vi "Calibrator Panel.vi"(8 "error in (no error)":errorcluster, 11 "Varian Magnet.lvclass In":refnum<class "Varian Magnet.lvclass">) -> (0 "error out":errorcluster, 3 "Varian Magnet.lvclass Out":refnum<class "Varian Magnet.lvclass">)   [LabVIEW 2009, in "Varian Magnet.lvclass"]
doc: "This is a low level control panel for the Varian magnet. It allows for reading and setting of the control voltage and displays the raw hall voltage. It also contains functions for calibrating various features of the magnet program."
uses:
  Varian Magnet.lvclass
  <vilib>/gmath/interp.llb/in_piecewise interp poly control.ctl
  Varian Magnet.lvclass/Varian Magnet.ctl
  <vilib>/Utility/file.llb/Write To Spreadsheet File (DBL).vi
  Varian/Varian.lvlib
  Fluke Multimeter/Fluke Multimeter.lvclass
  <vilib>/gmath/NI_Gmath.lvlib
panel:
  out "extrapolated":T1 {"x locations" format="%.4g"; "coefficients" format="%.4g"}
  in  "Write Current Calibration\nto Long-Term Calibration":bool
  in  "base volts":dbl=8.5
  in  "volt increment":dbl=-0.1
  in  "Max Field":dbl[unit]=0.8
  in  "Dwell Time (ms)":u32=1000
  in  "Calibrate Field":bool
  in  "Update Hall\nCalibration\nCoefficients":bool
  in  "Export Table":bool
  in  "Reset Table":bool
  in  "Hall Probe Calibration Table":dbl[][](array[numeric])
  in  "Save Point":bool
  out "Tesla":dbl
  in  "Gauss":dbl
  in  "Set Control Voltage":bool
  out "Current Field\nCalibration":cluster{dbl[], dbl[]}(graph)
  out "Hall Probe Voltage":dbl
  out "Control V":dbl
  in  "Set Control V":dbl
  in  "Copy Actual to Set":bool
  in  "Read Voltages":bool
  in  "stop":bool
  # "Long-Term Field\nCalibration"
  # "Hall Probe\nCalibration"
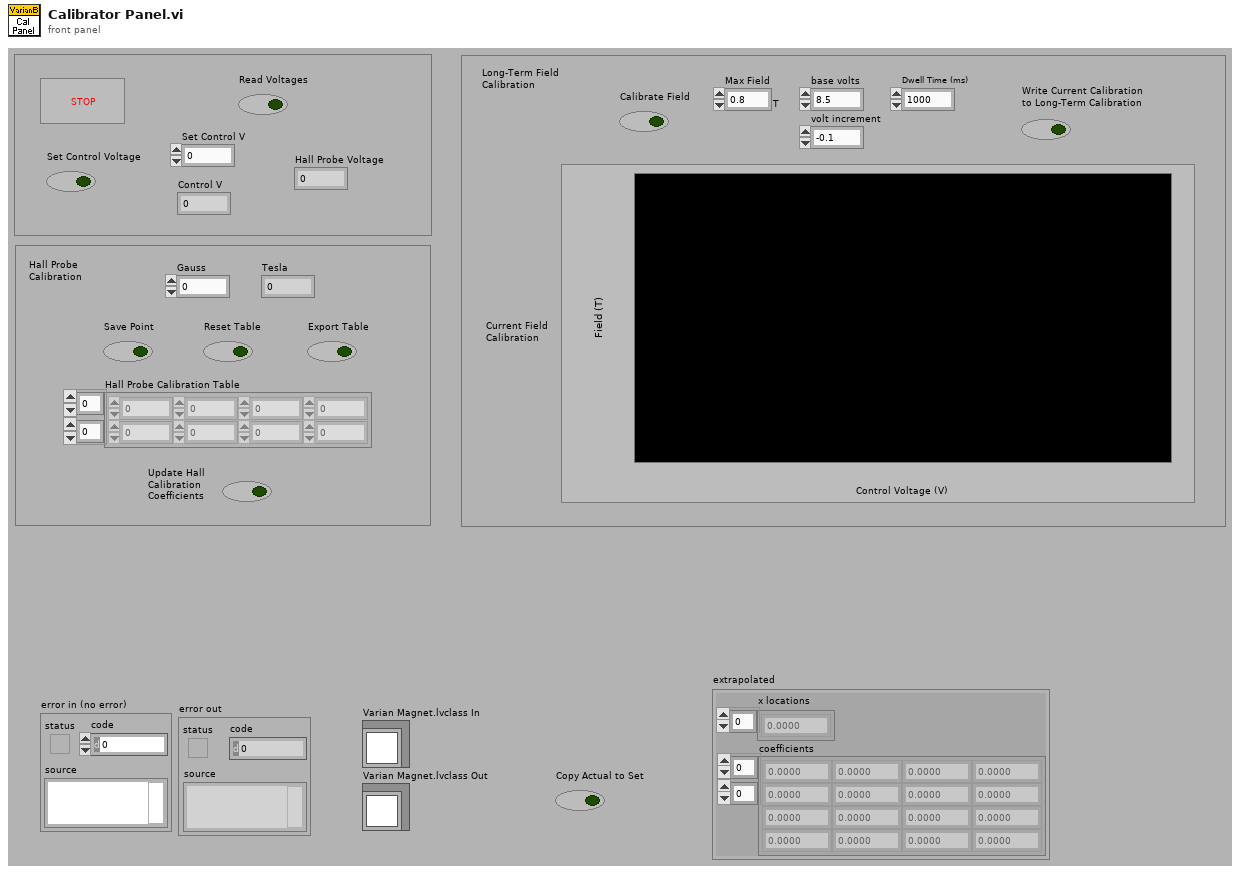
[diagram p1: front panel]
types:
  T1 = typedef "NI_Gmath.lvlib/in_piecewise interp poly control.ctl" = cluster{"x locations":dbl[], "coefficients":dbl[][]}
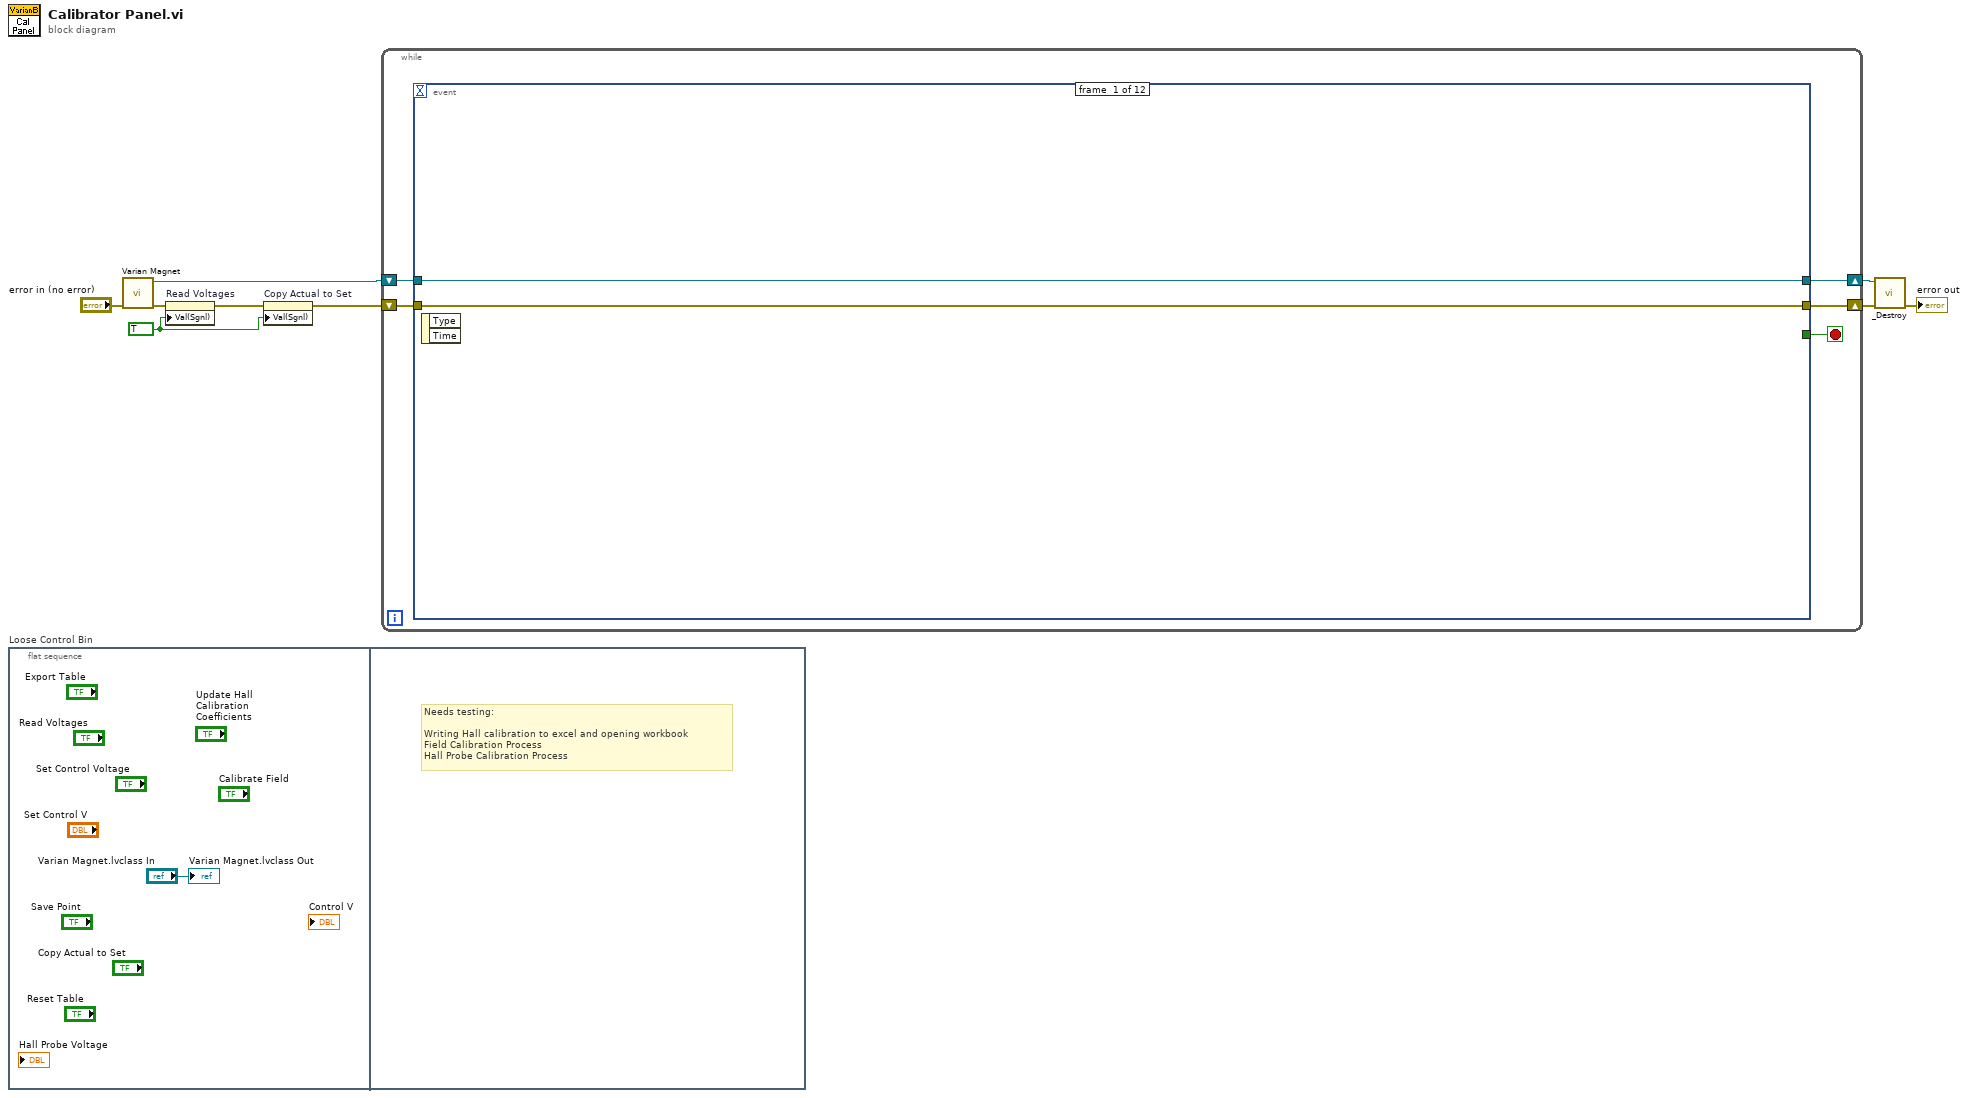
[diagram p0: block diagram]
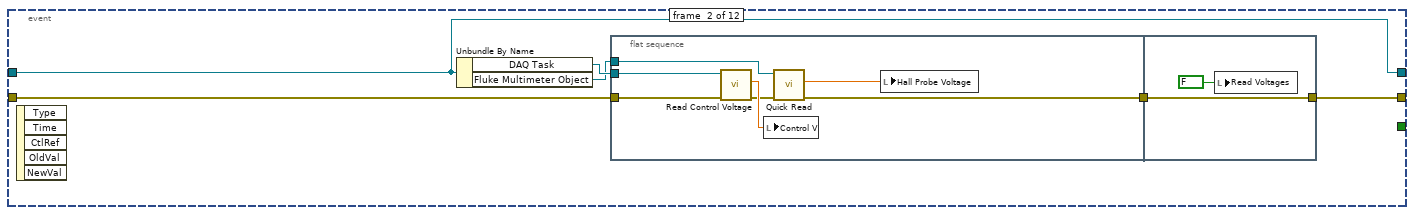
[diagram p2: hidden frame]
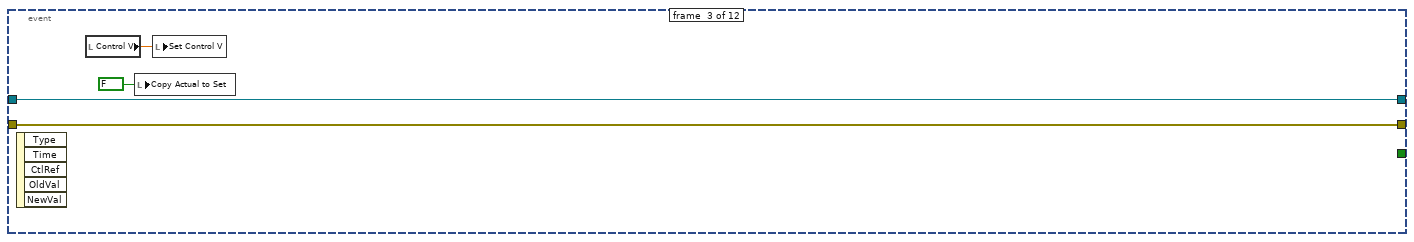
[diagram p3: hidden frame]
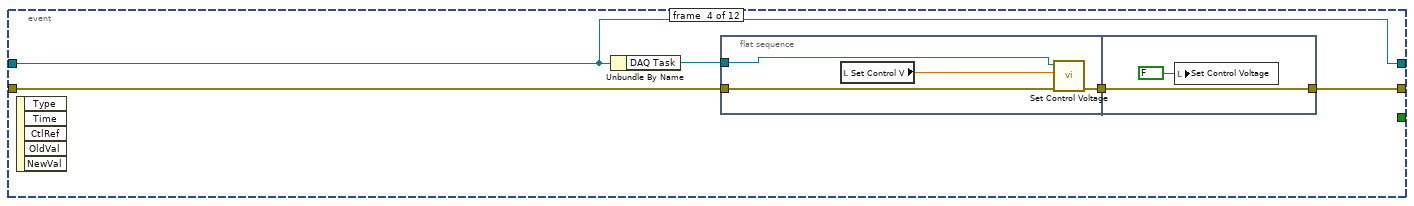
[diagram p4: hidden frame]
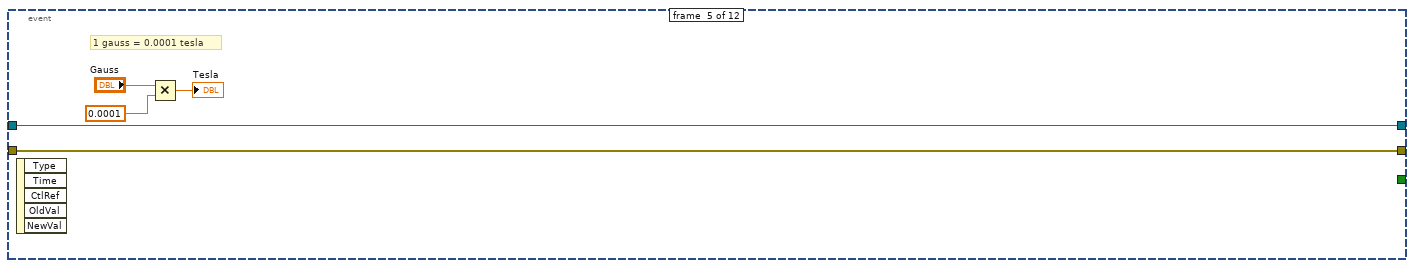
[diagram p5: hidden frame]
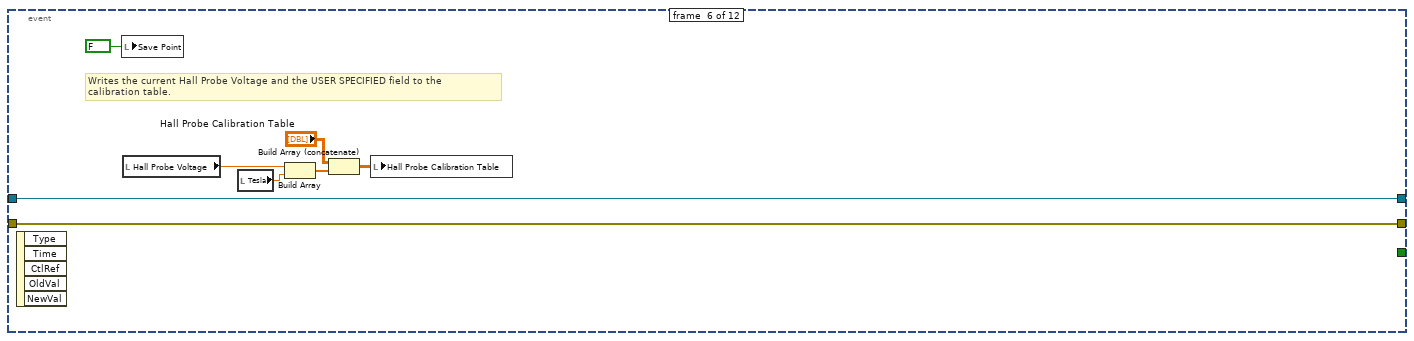
[diagram p6: hidden frame]
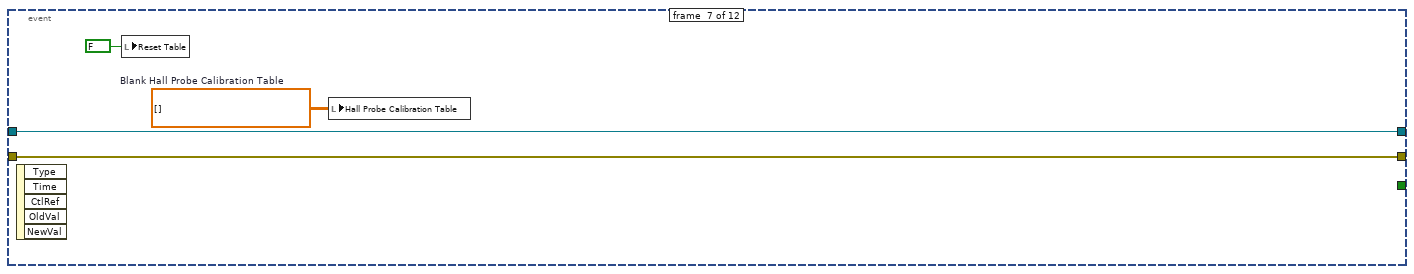
[diagram p7: hidden frame]
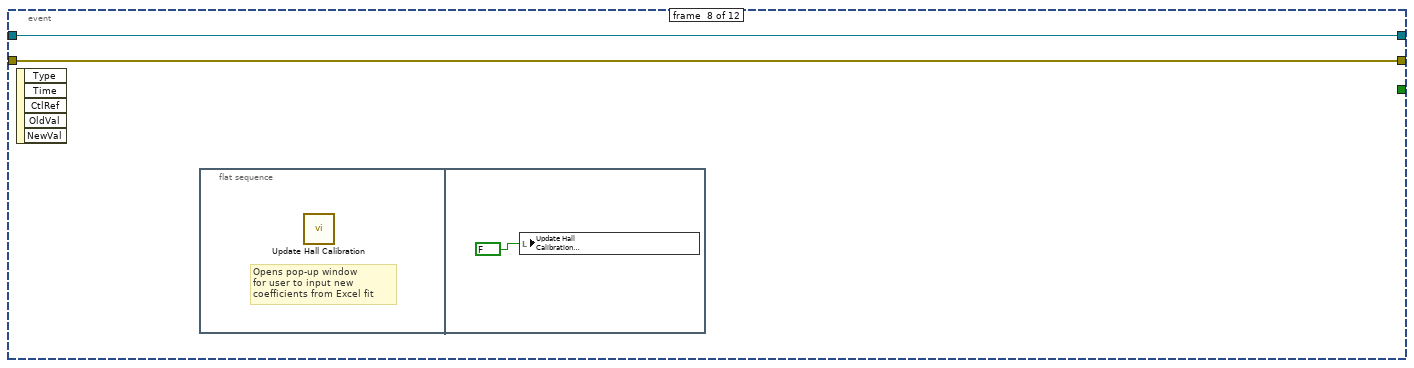
[diagram p8: hidden frame]
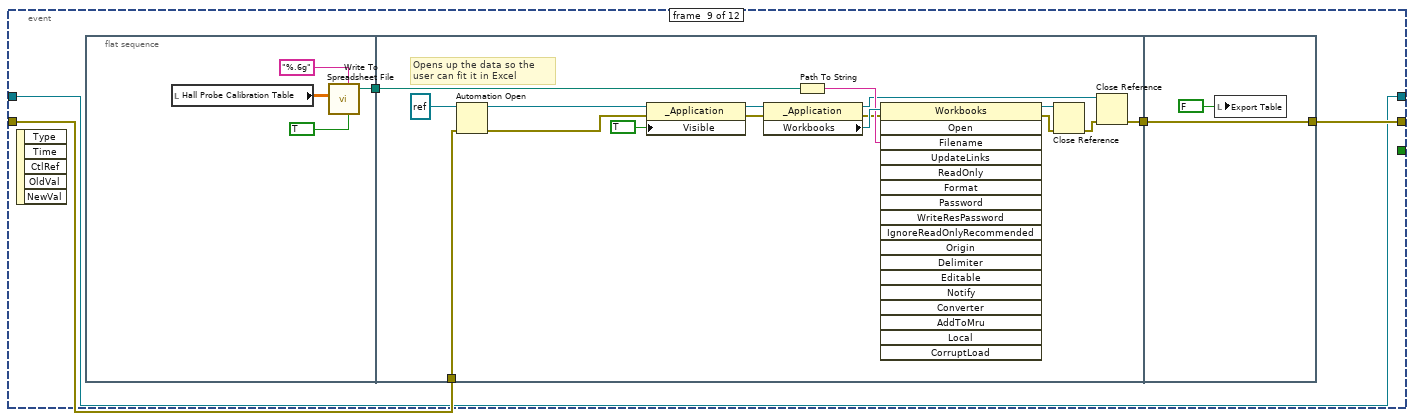
[diagram p9: hidden frame]
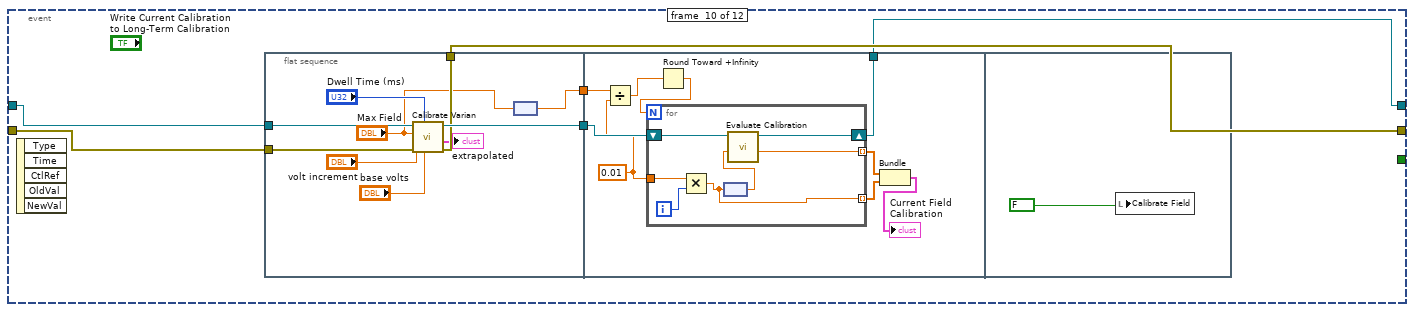
[diagram p10: hidden frame]
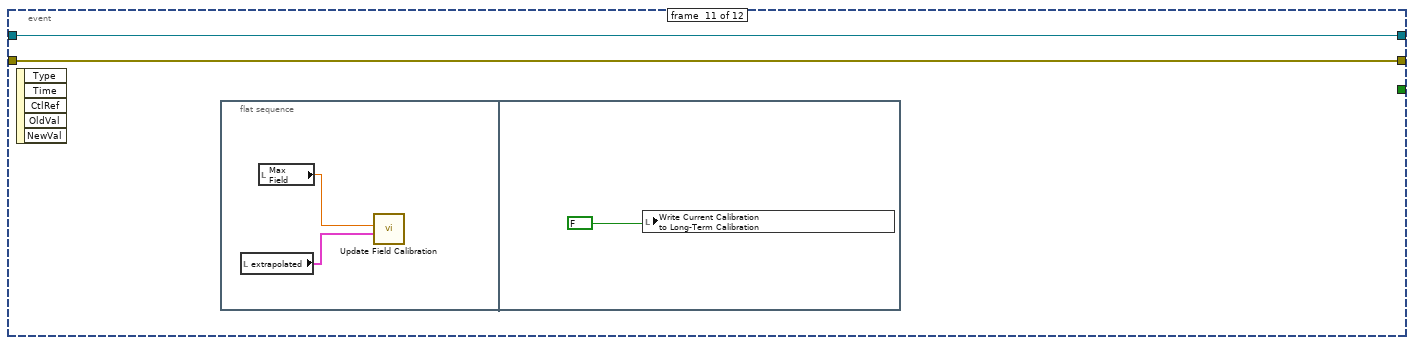
[diagram p11: hidden frame]
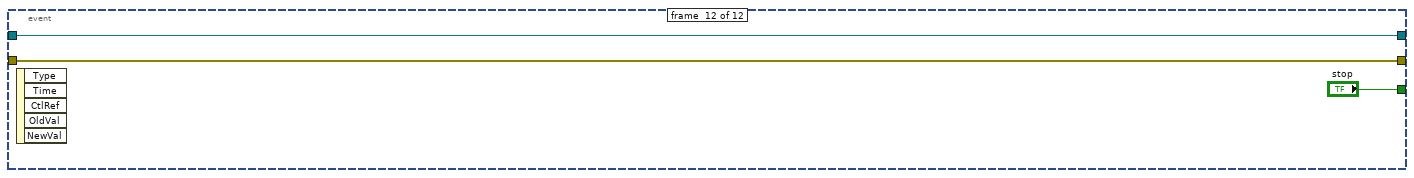
[diagram p12: hidden frame]
diagram:
  w1 = TRUE
  n1 = flat-sequence "Loose Control Bin" {
    frame #0 {
      "Varian Magnet.lvclass Out" <- "Varian Magnet.lvclass In"
    }
    frame #1 {
      # "Needs testing:\n\nWriting Hall calibration to excel and opening workbook\nField Calibration Process\nHall Probe Calibration Process"
    }
  }
  n2 = call "Varian Magnet.vi"("error in (no error)"="error in (no error)") -> ("error out"=w4:errorcluster, "Varian Magnet out"=w8:refnum<class "Varian Magnet.lvclass">)  [unwired: 9 in]
  n3 = property on="Read Voltages" class="Bool (strict)"(error in=w4, "Val(Sgnl)"=w1) -> (error out=w3:errorcluster)  [unwired: 1 in, 1 out]
  n4 = property on="Copy Actual to Set" class="Bool (strict)"(error in=w3, "Val(Sgnl)"=w1) -> (error out=w2:errorcluster)  [unwired: 1 in, 1 out]
  n5 = while {
    shift-right: [w14] -> w6
    shift-left: w2 -> [w13]
    shift-right: [w12] -> w7
    shift-left: w8 -> [w11]
    stop <- w15 stop-if-true
    n6 = event shown="[11] \"stop\": Value Change" {
      selector: _ -> [_ _ _ _ _ _ _ _ _ _ _ _]
      dyn-events: _ -> [_ _ _ _ _ _ _ _ _ _ _ _]
      timeout: _ -> [_ _ _ _ _ _ _ _ _ _ _ _]
      tunnel: [_ _ _ _ _ _ _ _ _ _ _ "stop"] -> w15
      tunnel: [w17 w19 w36 w38 w49 w53 w62 w65 w70 w99 w128 w134] -> w14
      tunnel: w13 -> [w17 w21 w36 w41 w49 w53 w62 w65 w72 w100 w128 w134]
      tunnel: [w16 w23 w35 w39 w48 w54 w61 w66 w68 w96 w129 w133] -> w12
      tunnel: w11 -> [w16 w23 w35 w39 w48 w54 w61 w66 w68 w98 w129 w133]
      event #0 {
        n7 = event-data() -> ()  [unwired: 1 in, 2 out]
      }
      event #1 {
        n8 = event-data() -> ()  [unwired: 1 in, 5 out]
        n9 = Unbundle By Name(w23) -> ("DAQ Task"=w22:refnum<k21>, "Fluke Multimeter Object"=w20:refnum<class "Fluke Multimeter.lvclass">)
        n10 = flat-sequence {
          tunnel: w22 -> [w30]
          tunnel: w21 -> [w29]
          tunnel: w20 -> [w27]
          tunnel: [w25] -> w18
          tunnel: [w32] -> w19
          tunnel: w18 -> [w32]
          frame #0 {
            n11 = call "Read Control Voltage.vi"("error in"=w29, "task in"=w30) -> ("error out"=w26:errorcluster, "Current Control Voltage"=w28:dbl)  [unwired: 7 in, 1 out]
            n12 = local write "Control V"(w28) -> ()
            n13 = call "Quick Read.vi"("error in (no error)"=w26, "Fluke Multimeter.lvclass In"=w27) -> ("error out"=w25:errorcluster, "measurement"=w24:dbl)  [unwired: 6 in, 2 out]
            n14 = local write "Hall Probe Voltage"(w24) -> ()
          }
          frame #1 {
            n15 = local write "Read Voltages"(FALSE) -> ()
          }
        }
      }
      event #2 {
        n16 = event-data() -> ()  [unwired: 1 in, 5 out]
        n17 = local read "Control V"() -> (w34:dbl)
        n18 = local write "Copy Actual to Set"(FALSE) -> ()
        n19 = local write "Set Control V"(w34) -> ()
      }
      event #3 {
        n20 = event-data() -> ()  [unwired: 1 in, 5 out]
        n21 = Unbundle By Name(w39) -> ("DAQ Task"=w40:refnum<k21>)
        n22 = flat-sequence {
          tunnel: w41 -> [w45]
          tunnel: w40 -> [w44]
          tunnel: [w42] -> w37
          tunnel: [w47] -> w38
          tunnel: w37 -> [w47]
          frame #0 {
            n23 = local read "Set Control V"() -> (w43:dbl)
            n24 = call "Set Control Voltage.vi"("error in"=w45, "Control Voltage"=w43, "task in"=w44) -> ("error out"=w42:errorcluster)  [unwired: 7 in, 1 out]
          }
          frame #1 {
            n25 = local write "Set Control Voltage"(FALSE) -> ()
          }
        }
      }
      event #4 {
        # "1 gauss = 0.0001 tesla"
        n26 = event-data() -> ()  [unwired: 1 in, 5 out]
        n27 = Multiply(x="Gauss", y=0.0001) -> (x*y=→"Tesla":dbl)
      }
      event #5 {
        # "Writes the current Hall Probe Voltage and the USER SPECIFIED field to the\ncalibration table."
        n28 = event-data() -> ()  [unwired: 1 in, 5 out]
        n29 = local write "Save Point"(FALSE) -> ()
        n30 = local read "Hall Probe Voltage"() -> (w59:dbl)
        n31 = local read "Tesla"() -> (w58:dbl)
        n32 = Build Array(w59, w58) -> (w57:dbl[])
        n33 = Build Array (concatenate)("Hall Probe Calibration Table", w57) -> (w56:dbl[][])
        n34 = local write "Hall Probe Calibration Table"(w56) -> ()
      }
      event #6 {
        w64 = dbl[][] []  # Blank Hall Probe Calibration Table
        n35 = event-data() -> ()  [unwired: 1 in, 5 out]
        n36 = local write "Reset Table"(FALSE) -> ()
        n37 = local write "Hall Probe Calibration Table"(w64) -> ()
      }
      event #7 {
        n38 = event-data() -> ()  [unwired: 1 in, 5 out]
        n39 = flat-sequence {
          frame #0 {
            # "Opens pop-up window\nfor user to input new\ncoefficients from Excel fit"
            n40 = call "Update Hall Calibration.vi"() -> ()  [unwired: 12 in]
          }
          frame #1 {
            n41 = local write "Update Hall\nCalibration\nCoefficients"(FALSE) -> ()
          }
        }
      }
      event #8 {
        n42 = event-data() -> ()  [unwired: 1 in, 5 out]
        n43 = flat-sequence {
          tunnel: [w73] -> w71
          tunnel: w72 -> [w92]
          tunnel: w71 -> [w87]
          tunnel: [w79] -> w69
          tunnel: [w94] -> w70
          tunnel: w69 -> [w94]
          frame #0 {
            n44 = local read "Hall Probe Calibration Table"() -> (w74:dbl[][])
            n45 = call-poly <vilib>:"Write To Spreadsheet File.vi"("transpose? (no:F)"=TRUE, "format (%.3f)"="%.6g", "2D data"=w74) -> ("new file path (Not A Path if cancelled)"=w73:path)  [unwired: 5 in]
          }
          frame #1 {
            # "Opens up the data so the\nuser can fit it in Excel"
            n46 = Automation Open(error in (no error)=w92, Automation Refnum=refnum<k7> refnum ("Excel Application")) -> (Automation Refnum=w90:refnum<k7>, error out=w85:errorcluster)  [unwired: 2 in]
            n47 = property class="_Application"(reference=w90, error in=w85, "Visible"=TRUE) -> (reference out=w82:refnum<k7>, error out=w84:errorcluster)
            n48 = property class="_Application"(reference=w82, error in=w84) -> (reference out=w77:refnum<k7>, error out=w83:errorcluster, "Workbooks"=w88:refnum<k7>)
            n49 = Path To String(path=w87) -> (string=w86:string)
            n50 = invoke class="Workbooks" method="Open"(reference=w88, error in=w83, "Filename"=w86) -> (reference out=w78:refnum<k7>, error out=w81:errorcluster)  [unwired: 15 in, 16 out]
            n51 = Close Reference(reference=w78, error in (no error)=w81) -> (error out=w80:errorcluster)
            n52 = Close Reference(reference=w77, error in (no error)=w80) -> (error out=w79:errorcluster)
          }
          frame #2 {
            n53 = local write "Export Table"(FALSE) -> ()
          }
        }
      }
      event #9 {
        n54 = event-data() -> ()  [unwired: 1 in, 5 out]
        n55 = flat-sequence {
          tunnel: w100 -> [w110]
          tunnel: [w104] -> w99
          tunnel: w98 -> [w109]
          tunnel: [w105] -> w97
          tunnel: [w102] -> w95
          tunnel: w97 -> [w119]
          tunnel: [w118] -> w96
          tunnel: w95 -> [w114]
          frame #0 {
            n56 = call "Calibrate Varian.vi"("base volts"="base volts", "Dwell Time (ms)"="Dwell Time (ms)", "error in"=w110, "volt increment"="volt increment", "Max Field"="Max Field", "varian in"=w109) -> ("error out"=w104:errorcluster, "extrapolated"=→"extrapolated":T1, "varian out"=w105:refnum<class "Varian Magnet.lvclass">)  [unwired: 3 in]
            n57 = node("Max Field") -> (w102:dbl)
          }
          frame #1 {
            w113 = 0.01 ("x")
            n58 = Divide(x=w114, y=w113) -> (x/y=w112:dbl)
            n59 = Round Toward +Infinity(x=w112) -> (ceil(x): smallest int >= x=w111:dbl)
            n60 = for {
              N: w111 -> [_]
              shift-right: [w125] -> w118
              shift-left: w119 -> [w126]
              tunnel: [w120] -> w116 mode=indexing
              tunnel: [w122] -> w117 mode=indexing
              tunnel: w113 -> [w121]
              i -> [w124]
              n61 = Multiply(x=w121, y=w124) -> (x*y=w120:dbl)
              n62 = node(w120) -> (w123:dbl[unit])
              n63 = call "Evaluate Calibration.vi"("tesla"=w123, "varian in"=w126) -> ("control voltage"=w122:dbl, "varian out"=w125:refnum<class "Varian Magnet.lvclass">)  [unwired: 8 in]
            }
            n64 = Bundle(w117, w116) -> (→"Current Field\nCalibration":cluster{dbl[], dbl[]})  [unwired: 1 in]
          }
          frame #2 {
            n65 = local write "Calibrate Field"(FALSE) -> ()
          }
        }
      }
      event #10 {
        n66 = event-data() -> ()  [unwired: 1 in, 5 out]
        n67 = flat-sequence {
          frame #0 {
            n68 = local read "extrapolated"() -> (w130:T1)
            n69 = local read "Max Field"() -> (w131:dbl[unit])
            n70 = call "Update Field Calibration.vi"("New Field Calibration"=w130, "Max Field"=w131) -> ()  [unwired: 10 in]
          }
          frame #1 {
            n71 = local write "Write Current Calibration\nto Long-Term Calibration"(FALSE) -> ()
          }
        }
      }
      event #11 {
        n72 = event-data() -> ()  [unwired: 1 in, 5 out]
      }
    }
  }
  n73 = call-dynamic "_Destroy.vi"("error in (no error)"=w6, "Instrument in"=w7) -> ("error out"=→"error out":errorcluster)  [unwired: 9 in]
